vi "ArrayDevCurveNames.vi"(0 "Experiment.lvclass In":refnum<class "Experiment.lvclass">, 5 "IndCourbe":i64 caption="Numéro de Balayage", 9 "NomDon":string[](array[string])=["RTêta;", "X&Y;"], 11 "error in":errorcluster) -> (4 "Exp.lvclass Out":refnum<class "Experiment.lvclass">, 6 "Scan list":string[](array[string]), 8 "VarPar list":string[](array[string]), 13 "CalcQIndex":cluster{"Tableau":i32[]}[](array[cluster]), 14 "DataQIndex":cluster{"Tableau":i32[]}[](array[cluster]), 15 "error out":errorcluster)   [LabVIEW 2019, in "Experiment.lvclass"]
doc: "Ce Vi créer la ligne d'entête du fichier texte de sauvegarde à partir du nombre de courbe voulu."
uses:
  Experiment.lvclass
  Experiment.lvclass/Experiment.ctl
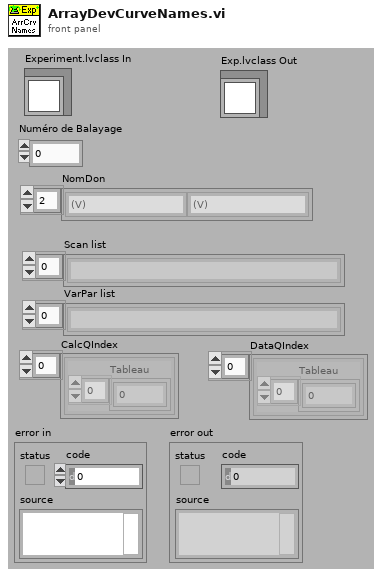
[diagram p1: front panel]
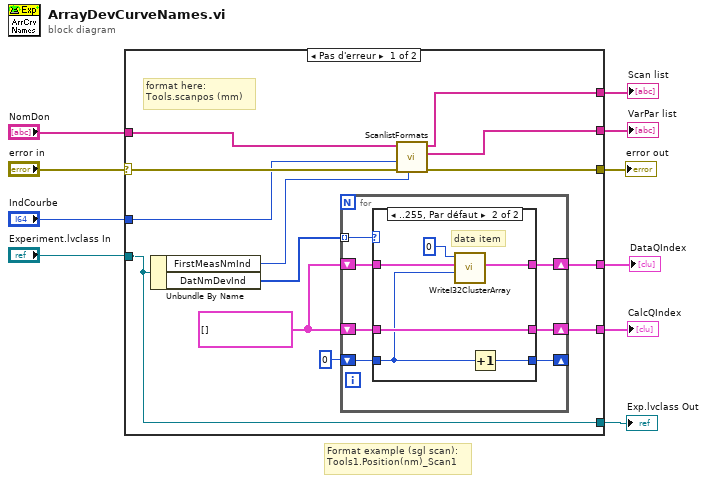
[diagram p0: block diagram]
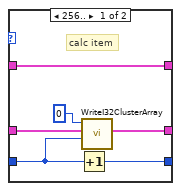
[diagram p2: hidden frame]
diagram:
  # "Format example (sgl scan):\nTools1.Position(nm)_Scan1"
  n1 = case shown="Pas d'erreur" "error in" {
    selector: "error in" -> [w14 w44]
    tunnel: [w13 w44] -> w9
    tunnel: [w16 _] -> w8
    tunnel: "NomDon" -> [w17 _]
    tunnel: "Experiment.lvclass In" -> [w23 w43]
    tunnel: "IndCourbe" -> [w11 _]
    tunnel: [w23 w43] -> w4
    tunnel: [w20 _] -> w3
    tunnel: [w19 _] -> w2
    tunnel: [w15 _] -> w1
    frame No Error {
      w21 = cluster{"Tableau":i32[]}[] [] ("CalcQIndex")
      # "format here:\nTools.scanpos (mm)"
      n2 = Unbundle By Name(w23) -> ("FirstMeasNmInd"=w12:i32, "DatNmDevInd"=w22:i32[])
      n3 = for {
        tunnel: w22 -> [w30] mode=indexing
        shift-right: [w27] -> w19
        shift-left: w21 -> [w26]
        shift-right: [w28] -> w20
        shift-left: w21 -> [w29]
        shift-right: [w24] -> _
        shift-left: 0 ("Data") -> [w25]
        n4 = case shown="..255, Par défaut" w30 {
          tunnel: w29 -> [w36 w42]
          tunnel: [w35 w42] -> w28
          tunnel: w25 -> [w32 w38]
          tunnel: [w33 w39] -> w27
          tunnel: w26 -> [w33 w40]
          tunnel: [w31 w37] -> w24
          frame 256.. {
            # "calc item"
            n5 = Increment(x=w32) -> (x+1=w31:i32)
            n6 = call <userlib>:"WriteI32ClusterArray.vi"("Data"=w32, "array"=w36, "ClusterInd"=0) -> ("output array"=w35:cluster{"Tableau":i32[]}[])  [unwired: 7 in, 1 out]
          }
          frame ..255, Default {
            # "data item"
            n7 = call <userlib>:"WriteI32ClusterArray.vi"("Data"=w38, "array"=w40, "ClusterInd"=0) -> ("output array"=w39:cluster{"Tableau":i32[]}[])  [unwired: 7 in, 1 out]
            n8 = Increment(x=w38) -> (x+1=w37:i32)
          }
        }
      }
      n9 = call "ScanlistFormats.vi"("FirstMeasNmInd"=w12, "ErrorIn(No Error)"=w14, "IndCourbe"=w11, "DatNmArr"=w17) -> ("Err Out"=w13:errorcluster, "VarParList"=w15:string[], "ScanList"=w16:string[])  [unwired: 5 in]
    }
    frame Error {
    }
  }
  "error out" <- w9
  "Scan list" <- w8
  "Exp.lvclass Out" <- w4
  "CalcQIndex" <- w3
  "DataQIndex" <- w2
  "VarPar list" <- w1
